vi "Initialize AI Task.vi"(8 "error in (no error)":errorcluster, 11 "BNT_ULx-MCSV in":refnum<class "BNT_ULx-MCSV.lvclass">) -> (0 "error out":errorcluster, 3 "AI ULx Task":refnum<k24>)   [LabVIEW 2021, in "BNT_ULx.lvlib" / "BNT_ULx-MCSV.lvclass"]
doc: "Initialize ULx Analog Input task. Every derived class needs to start the task on its own.\n\n<b>Default Implementation:</b> Analog Input Voltage\n\nThis dynamic dispatch VI can be overritten by derived classes to implement other analog input tasks."
uses:
  BNT_ULx-MCSV.lvclass
  <vilib>/ULx/ULx_LV.dll
  BNT_ULx-MCSV.lvclass/BNT_ULx-MCSV.ctl
  <vilib>/ULx/Create Channel.llb/ULx Create Channel (AI-Voltage-Basic).vi
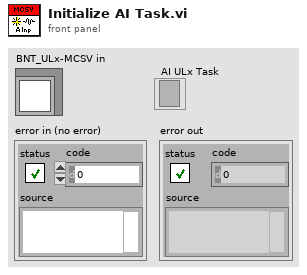
[diagram p1: front panel]
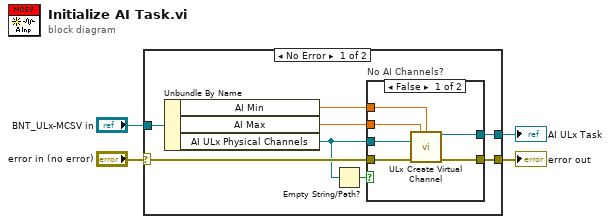
[diagram p0: block diagram]
diagram:
  n1 = case shown="No Error" "error in (no error)" {
    selector: "error in (no error)" -> [w9 w20]
    tunnel: [w10 w20] -> w3
    tunnel: "BNT_ULx-MCSV in" -> [w5 _]
    tunnel: [w6 _] -> w1
    frame No Error {
      n2 = Unbundle By Name(w5) -> ("AI Min"=w12:dbl, "AI Max"=w11:dbl, "AI ULx Physical Channels"=w7:refnum<k21>)
      n3 = Empty String/Path?(string/path=w7) -> (empty?=w8:bool)
      n4 = case "No AI Channels?" shown="False" w8 {
        tunnel: w7 -> [w14 _]
        tunnel: w12 -> [w15 _]
        tunnel: w11 -> [w16 _]
        tunnel: [w17 w19] -> w10
        tunnel: w9 -> [w18 w19]
        tunnel: [w13 _] -> w6
        frame False {
          n5 = call-poly <vilib>:"ULx Create Virtual Channel.vi"("maximum value"=w16, "minimum value"=w15, "physical channels"=w14, "error in"=w18) -> ("task out"=w13:refnum<k24>, "error out"=w17:errorcluster)  [unwired: 10 in]
        }
        frame True {
        }
      }
    }
    frame Error {
    }
  }
  "error out" <- w3
  "AI ULx Task" <- w1
